vi "MC - String To Date.vi"(0 "String Date":string) -> (1 "Month":u32, 2 "Day":u32, 3 "Year":u32)   [LabVIEW 2015]
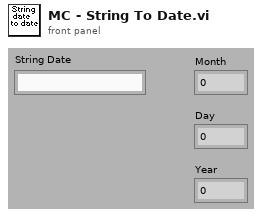
[diagram p1: front panel]
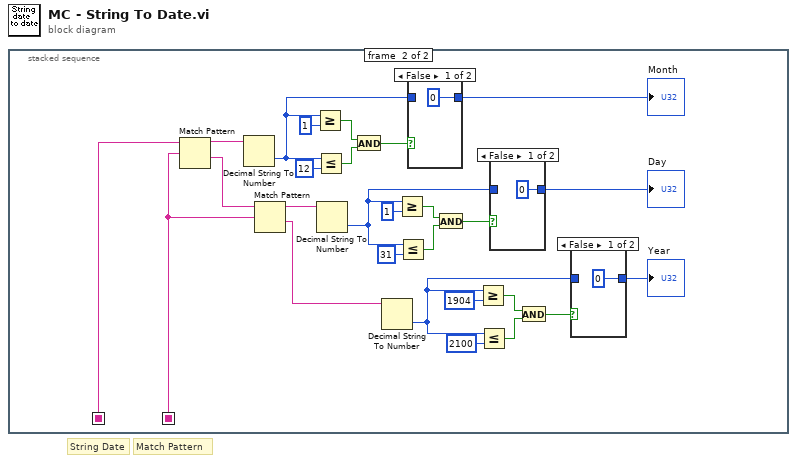
[diagram p0: block diagram]
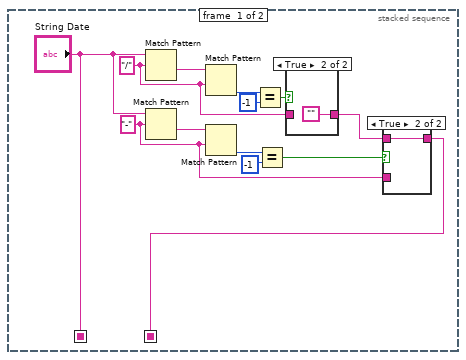
[diagram p2: hidden frame]
diagram:
  # "Match Pattern"
  # "String Date"
  n1 = stacked-sequence {
    seq-local: ["String Date" _] -> [_ w19]
    seq-local: [w1 _] -> [_ w18]
    frame #0 {
      w4 = "-" ("regular expression")
      w5 = "/" ("regular expression")
      n2 = Match Pattern(string="String Date", regular expression=w5) -> (after substring=w7:string)  [unwired: 4 out]
      n3 = Match Pattern(string="String Date", regular expression=w4) -> (after substring=w9:string)  [unwired: 4 out]
      n4 = Match Pattern(string=w7, regular expression=w5) -> (offset past match=w6:i32)  [unwired: 1 in, 3 out]
      n5 = Match Pattern(string=w9, regular expression=w4) -> (offset past match=w8:i32)  [unwired: 4 out]
      n6 = Equal?(x=w6, y=-1) -> (x = y?=w11:bool)
      n7 = Equal?(x=w8, y=-1) -> (x = y?=w10:bool)
      n8 = case shown="True" w11 {
        tunnel: w5 -> [w16 _]
        tunnel: [w16 ""] -> w3
        frame False {
        }
        frame True {
        }
      }
      n9 = case shown="True" w10 {
        tunnel: w4 -> [w14 _]
        tunnel: w3 -> [_ w15]
        tunnel: [w14 w15] -> w1
        frame False {
        }
        frame True {
        }
      }
    }
    frame #1 {
      n10 = Match Pattern(string=w19, regular expression=w18) -> (before substring=w35:string, after substring=w23:string)  [unwired: 3 out]
      n11 = Decimal String To Number(string=w35) -> (number=w26:i32)  [unwired: 3 out]
      n12 = Match Pattern(string=w23, regular expression=w18) -> (before substring=w36:string, after substring=w37:string)  [unwired: 3 out]
      n13 = Greater Or Equal?(x=w26, y=1) -> (x >= y?=w38:bool)
      n14 = Less Or Equal?(x=w26, y=12) -> (x <= y?=w39:bool)
      n15 = Decimal String To Number(string=w36) -> (number=w33:i32)  [unwired: 3 out]
      n16 = And(x=w38, y=w39) -> (x .and. y?=w40:bool)
      n17 = Decimal String To Number(string=w37) -> (number=w34:i32)  [unwired: 3 out]
      n18 = Greater Or Equal?(x=w33, y=1) -> (x >= y?=w43:bool)
      n19 = Less Or Equal?(x=w33, y=31) -> (x <= y?=w44:bool)
      n20 = case shown="False" w40 {
        tunnel: w26 -> [_ w50]
        tunnel: [0 w50] -> w22
        frame False {
        }
        frame True {
        }
      }
      "Month" <- w22
      n21 = And(x=w43, y=w44) -> (x .and. y?=w41:bool)
      n22 = Greater Or Equal?(x=w34, y=1904) -> (x >= y?=w32:bool)
      n23 = Less Or Equal?(x=w34, y=2100) -> (x <= y?=w31:bool)
      n24 = case shown="False" w41 {
        tunnel: w33 -> [_ w48]
        tunnel: [0 w48] -> w20
        frame False {
        }
        frame True {
        }
      }
      "Day" <- w20
      n25 = And(x=w32, y=w31) -> (x .and. y?=w42:bool)
      n26 = case shown="False" w42 {
        tunnel: w34 -> [_ w46]
        tunnel: [0 w46] -> w21
        frame False {
        }
        frame True {
        }
      }
      "Year" <- w21
    }
  }
